vi "JKI Python Bridge - Example 2 Nodes.vi"() -> ()   [LabVIEW 2020]
uses:
  Server/Server.lvclass
  Call/Call.lvclass
  Server/Register for Events (Single PyObject).vi
  Server/Type Definitions/Python Method.ctl
  3cf1a9b7-339d-49c1-9244-9fdeeda8039a.vi
  c3fdb256-908c-4137-97ff-72e1cc020f62.vi
  947fcaa3-6c5b-4cf2-b114-889b666fad60.vi
  09dd4288-c2f4-46fd-9205-16318354609d.vi
panel:
  out "Number of Connections":u32
  out "Client Connected":bool
  out "error out":errorcluster
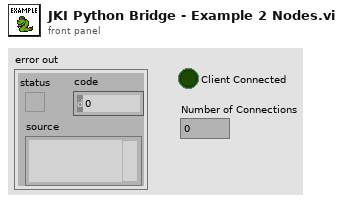
[diagram p1: front panel]
types:
  T1 = typedef "jki_python_bridge.lvlib/Server.lvclass/Python Method.ctl" = cluster{"Name":string, "Arguments":string[], "Documentation":string}
  T2 = typedef "jki_python_bridge.lvlib/Server.lvclass/Python Method Call - Event Registration.ctl" = refnum<event-registration>
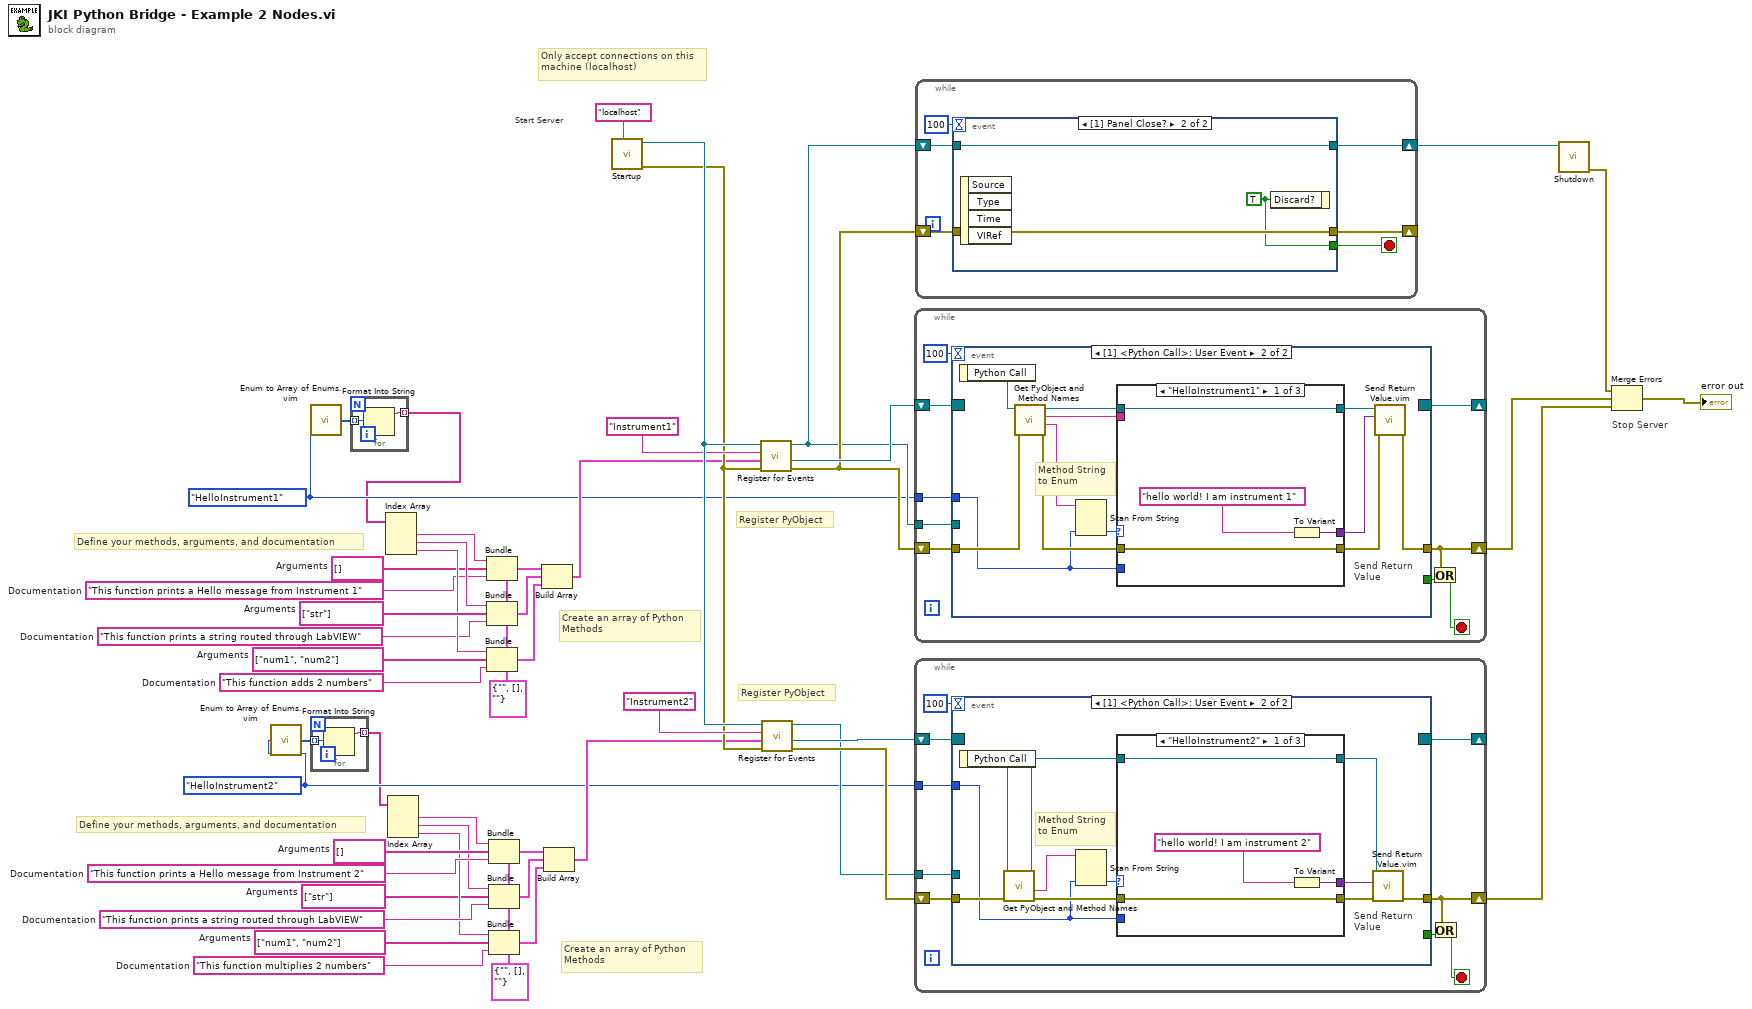
[diagram p0: block diagram]
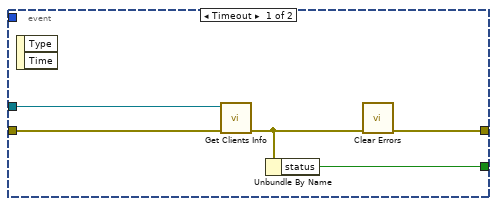
[diagram p2: hidden frame]
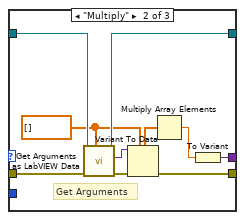
[diagram p3: hidden frame]
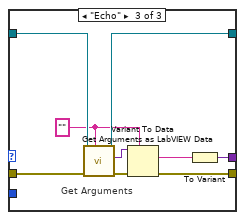
[diagram p4: hidden frame]
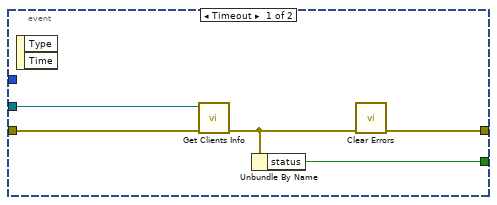
[diagram p5: hidden frame]
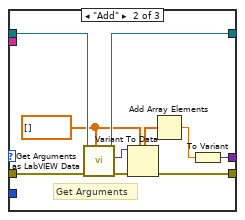
[diagram p6: hidden frame]
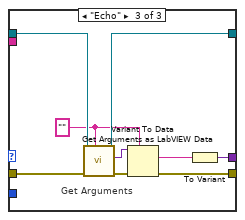
[diagram p7: hidden frame]
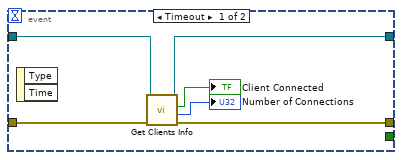
[diagram p8: hidden frame]
diagram:
  w20 = string[] []  # Arguments
  w19 = T1 {"Name"="", "Arguments"=[], "Documentation"=""} ("Method")
  w18 = "This function multiplies 2 numbers"  # Documentation
  w17 = "This function prints a string routed through LabVIEW"  # Documentation
  w16 = "This function prints a Hello message from Instrument 2"  # Documentation
  w11 = string[] ["num1", "num2"]  # Arguments
  w10 = string[] ["str"]  # Arguments
  w22 = string[] []  # Arguments
  w23 = T1 {"Name"="", "Arguments"=[], "Documentation"=""} ("Method")
  w24 = "This function adds 2 numbers"  # Documentation
  w25 = "This function prints a string routed through LabVIEW"  # Documentation
  w26 = "This function prints a Hello message from Instrument 1"  # Documentation
  w31 = string[] ["num1", "num2"]  # Arguments
  w32 = string[] ["str"]  # Arguments
  w2 = enum16{"HelloInstrument2", "Echo", "Multiply"}."HelloInstrument2"
  w5 = enum16{"HelloInstrument1", "Echo", "Add"}."HelloInstrument1"
  # "Create an array of Python \nMethods"
  # "Define your methods, arguments, and documentation"
  # "Create an array of Python \nMethods"
  # "Define your methods, arguments, and documentation"
  # "Register PyObject"
  # "Register PyObject"
  # "Stop Server"
  # "Start Server"
  # "Only accept connections on this machine (localhost)"
  n1 = call "Enum to Array of Enums.vim"("enum"=w2) -> ("array of enums"=w3:enum16{"HelloInstrument2", "Echo", "Multiply"}[])
  n2 = call "Enum to Array of Enums.vim"("enum"=w5) -> ("array of enums"=w6:enum16{"HelloInstrument1", "Echo", "Add"}[])
  n3 = for {
    tunnel: w3 -> [w52] mode=indexing
    tunnel: [w51] -> w1 mode=indexing
    n4 = Format Into String(w52) -> (resulting string=w51:string)  [unwired: 3 in, 1 out]
  }
  n5 = for {
    tunnel: w6 -> [w54] mode=indexing
    tunnel: [w53] -> w4 mode=indexing
    n6 = Format Into String(w54) -> (resulting string=w53:string)  [unwired: 3 in, 1 out]
  }
  n7 = Index Array(array=w4) -> (element #1=w34:string, element #2=w33:string, element #3=w30:string)  [unwired: 3 in]
  n8 = Index Array(array=w1) -> (element #1=w8:string, element #2=w9:string, element #3=w12:string)  [unwired: 3 in]
  n9 = Bundle(cluster=w23, "Name"=w34, "Arguments"=w22, "Documentation"=w26) -> (w29:T1)
  n10 = Bundle(cluster=w23, "Name"=w33, "Arguments"=w32, "Documentation"=w25) -> (w28:T1)
  n11 = Bundle(cluster=w23, "Name"=w30, "Arguments"=w31, "Documentation"=w24) -> (w27:T1)
  n12 = Bundle(cluster=w19, "Name"=w8, "Arguments"=w20, "Documentation"=w16) -> (w13:T1)
  n13 = Bundle(cluster=w19, "Name"=w9, "Arguments"=w10, "Documentation"=w17) -> (w14:T1)
  n14 = Bundle(cluster=w19, "Name"=w12, "Arguments"=w11, "Documentation"=w18) -> (w15:T1)
  n15 = Build Array(w29, w28, w27) -> (w21:T1[])
  n16 = Build Array(w13, w14, w15) -> (w7:T1[])
  n17 = call "Startup.vi"("IP Address (localhost)"="localhost" ("name")) -> ("error out"=w39:errorcluster, "JKI_Python_Server out"=w49:refnum<class "Server.lvclass">)  [unwired: 9 in]
  n18 = call-poly "Register for Events.vi"("error in (no error)"=w39, "Functions"=w21, "PyObject Name"="Instrument1" ("Python Node Name"), "JKI_Python_Server in"=w49) -> ("error out"=w42:errorcluster, "Python"=w43:T2, "JKI_Python_Server out"=w38:refnum<class "Server.lvclass">)  [unwired: 5 in]
  n19 = call-poly "Register for Events.vi"("error in (no error)"=w39, "Functions"=w7, "PyObject Name"="Instrument2" ("Python Node Name"), "JKI_Python_Server in"=w49) -> ("error out"=w45:errorcluster, "Python"=w44:T2, "JKI_Python_Server out"=w37:refnum<class "Server.lvclass">)  [unwired: 5 in]
  n20 = while {
    shift-right: [w57] -> w46
    shift-left: w42 -> [w62]
    shift-right: [w60] -> _
    shift-left: w43 -> [w63]
    tunnel: w5 -> [w59]
    tunnel: w38 -> [w58]
    stop <- w56 stop-if-true
    n21 = event shown="[1] <Python Call>: User Event" {
      selector: w63 -> [_ _]
      dyn-events: [_ _] -> w60
      timeout: 100 -> [_ _]
      tunnel: [w64 w73] -> w57
      tunnel: w62 -> [w68 w78]
      tunnel: w59 -> [_ w75]
      tunnel: w58 -> [w67 _]
      tunnel: [w65 _] -> w55
      event Timeout {
        n22 = event-data() -> ()  [unwired: 1 in, 2 out]
        n23 = call "Get Clients Info.vi"("error in (no error)"=w68, "JKI_Python_Server in"=w67) -> ("error out"=w66:errorcluster)  [unwired: 5 in, 4 out]
        n24 = Unbundle By Name(w66) -> ("status"=w65:bool)
        n25 = call <vilib>:"Clear Errors.vi"("error in (no error)"=w66) -> ("error out"=w64:errorcluster)  [unwired: 5 in, 1 out]
      }
      event User Event {
        # "Send Return\nValue"
        # "Method String to Enum"
        n26 = event-data() -> ("Python Call"=w79:refnum<class "Call.lvclass">)  [unwired: 1 in]
        n27 = call "Get PyObject and Method Names.vi"("error in (no error)"=w78, "Call in"=w79) -> ("error out"=w77:errorcluster, "Method Name"=w70:string, "PyObject Name"=w69:string, "Call out"=w76:refnum<class "Call.lvclass">)  [unwired: 5 in, 1 out]
        n28 = Scan From String(input string=w70, default 1=w75) -> (output 1=w80:enum16{"HelloInstrument1", "Echo", "Add"})  [unwired: 3 in, 3 out]
        n29 = case shown="\"HelloInstrument1\"" w80 {
          tunnel: [w81 w85 w95] -> w72
          tunnel: w77 -> [w83 w88 w99]
          tunnel: [w83 w93 w103] -> w74
          tunnel: [w82 w90 w101] -> w71
          tunnel: w76 -> [w82 w91 w102]
          tunnel: w75 -> [_ _ _]
          tunnel: w69 -> [_ _ _]
          frame "HelloInstrument1" {
            n30 = To Variant(anything="hello world! I am instrument 1" ("Arguments")) -> (Variant=w81:variant)
          }
          frame "Add" {
            w86 = dbl[] []
            # "Get Arguments"
            n31 = call "Get Arguments as LabVIEW Data.vi"("type"=w86, "error in (no error)"=w88, "Call in"=w91) -> ("error out"=w87:errorcluster, "LabVIEW Data"=w89:variant, "Call out"=w90:refnum<class "Call.lvclass">)  [unwired: 6 in]
            n32 = Variant To Data(error in=w87, type=w86, Variant=w89) -> (data=w94:dbl[], error out=w93:errorcluster)
            n33 = Add Array Elements(numeric array=w94) -> (sum=w92:dbl)
            n34 = To Variant(anything=w92) -> (Variant=w85:variant)
          }
          frame "Echo" {
            w97 = ""
            # "Get Arguments"
            n35 = call "Get Arguments as LabVIEW Data.vi"("type"=w97, "error in (no error)"=w99, "Call in"=w102) -> ("error out"=w98:errorcluster, "LabVIEW Data"=w100:variant, "Call out"=w101:refnum<class "Call.lvclass">)  [unwired: 6 in]
            n36 = Variant To Data(error in=w98, type=w97, Variant=w100) -> (data=w96:string, error out=w103:errorcluster)
            n37 = To Variant(anything=w96) -> (Variant=w95:variant)
          }
        }
        n38 = call "Send Return Value.vim"("error in (no error)"=w74, "Return Value"=w72, "Response in"=w71) -> ("error out"=w73:errorcluster)  [unwired: 8 in]
      }
    }
    n39 = Or(x=w57, y=w55) -> (x .or. y?=w56:bool)
  }
  n40 = while {
    shift-right: [w106] -> w47
    shift-left: w45 -> [w111]
    shift-right: [w109] -> _
    shift-left: w44 -> [w112]
    tunnel: w2 -> [w108]
    tunnel: w37 -> [w107]
    stop <- w105 stop-if-true
    n41 = event shown="[1] <Python Call>: User Event" {
      selector: w112 -> [_ _]
      dyn-events: [_ _] -> w109
      timeout: 100 -> [_ _]
      tunnel: [w113 w120] -> w106
      tunnel: w111 -> [w117 w126]
      tunnel: w108 -> [_ w123]
      tunnel: w107 -> [w116 _]
      tunnel: [w114 _] -> w104
      event Timeout {
        n42 = event-data() -> ()  [unwired: 1 in, 2 out]
        n43 = call "Get Clients Info.vi"("error in (no error)"=w117, "JKI_Python_Server in"=w116) -> ("error out"=w115:errorcluster)  [unwired: 5 in, 4 out]
        n44 = Unbundle By Name(w115) -> ("status"=w114:bool)
        n45 = call <vilib>:"Clear Errors.vi"("error in (no error)"=w115) -> ("error out"=w113:errorcluster)  [unwired: 5 in, 1 out]
      }
      event User Event {
        # "Send Return\nValue"
        # "Method String to Enum"
        n46 = event-data() -> ("Python Call"=w127:refnum<class "Call.lvclass">)  [unwired: 1 in]
        n47 = call "Get PyObject and Method Names.vi"("error in (no error)"=w126, "Call in"=w127) -> ("error out"=w125:errorcluster, "Method Name"=w122:string, "Call out"=w124:refnum<class "Call.lvclass">)  [unwired: 5 in, 2 out]
        n48 = Scan From String(input string=w122, default 1=w123) -> (output 1=w128:enum16{"HelloInstrument2", "Echo", "Multiply"})  [unwired: 3 in, 3 out]
        n49 = case shown="\"HelloInstrument2\"" w128 {
          tunnel: [w129 w133 w143] -> w119
          tunnel: w125 -> [w131 w136 w147]
          tunnel: [w131 w141 w151] -> w121
          tunnel: [w130 w138 w149] -> w118
          tunnel: w124 -> [w130 w139 w150]
          tunnel: w123 -> [_ _ _]
          frame "HelloInstrument2" {
            n50 = To Variant(anything="hello world! I am instrument 2" ("Arguments")) -> (Variant=w129:variant)
          }
          frame "Multiply" {
            w134 = dbl[] []
            # "Get Arguments"
            n51 = call "Get Arguments as LabVIEW Data.vi"("type"=w134, "error in (no error)"=w136, "Call in"=w139) -> ("error out"=w135:errorcluster, "LabVIEW Data"=w137:variant, "Call out"=w138:refnum<class "Call.lvclass">)  [unwired: 6 in]
            n52 = Variant To Data(error in=w135, type=w134, Variant=w137) -> (data=w142:dbl[], error out=w141:errorcluster)
            n53 = Multiply Array Elements(1:w142) -> (0:w140:dbl)
            n54 = To Variant(anything=w140) -> (Variant=w133:variant)
          }
          frame "Echo" {
            w145 = ""
            # "Get Arguments"
            n55 = call "Get Arguments as LabVIEW Data.vi"("type"=w145, "error in (no error)"=w147, "Call in"=w150) -> ("error out"=w146:errorcluster, "LabVIEW Data"=w148:variant, "Call out"=w149:refnum<class "Call.lvclass">)  [unwired: 6 in]
            n56 = Variant To Data(error in=w146, type=w145, Variant=w148) -> (data=w144:string, error out=w151:errorcluster)
            n57 = To Variant(anything=w144) -> (Variant=w143:variant)
          }
        }
        n58 = call "Send Return Value.vim"("error in (no error)"=w121, "Return Value"=w119, "Response in"=w118) -> ("error out"=w120:errorcluster)  [unwired: 8 in]
      }
    }
    n59 = Or(x=w106, y=w104) -> (x .or. y?=w105:bool)
  }
  n60 = while {
    shift-right: [w153] -> _
    shift-left: w42 -> [w157]
    shift-right: [w154] -> w48
    shift-left: w38 -> [w155]
    stop <- w152 stop-if-true
    n61 = event shown="[1] Panel Close?" {
      selector: _ -> [_ _]
      dyn-events: _ -> [_ _]
      timeout: 100 -> [_ _]
      tunnel: [w161 w166] -> w153
      tunnel: w157 -> [w162 w166]
      tunnel: w155 -> [w163 w165]
      tunnel: [w160 w165] -> w154
      tunnel: [_ w164] -> w152
      event Timeout {
        n62 = event-data() -> ()  [unwired: 1 in, 2 out]
        n63 = call "Get Clients Info.vi"("error in (no error)"=w162, "JKI_Python_Server in"=w163) -> ("error out"=w161:errorcluster, "Number of Connections"=→"Number of Connections":u32, "Client Connected"=→"Client Connected":bool, "JKI_Python_Server out"=w160:refnum<class "Server.lvclass">)  [unwired: 5 in, 1 out]
      }
      event Panel Close? {
        w164 = TRUE ("Discard?")
        n64 = event-data() -> ()  [unwired: 1 in, 4 out]
        n65 = event-data("Discard?"=w164) -> ()  [unwired: 1 in, 1 out]
      }
    }
  }
  n66 = call "Shutdown.vi"("JKI_Python_Server in"=w48) -> ("error out"=w36:errorcluster)  [unwired: 10 in]
  n67 = Merge Errors(w36, w46, w47) -> (→"error out":errorcluster)
